vi "CRYAPI WSYSTEM.vi"(8 "sData":string, 9 "pVIF":refnum<vi>, 10 "sOption":string, 11 "sAction":string) -> (0 "bResult":bool=TRUE, 1 "pVIF_Out":refnum<vi>, 2 "sData_Out":string, 3 "tFrame_Out":T2)   [LabVIEW 2013]
uses:
  <vilib>/Utility/miscctls.llb/LVRectTypeDef.ctl
  CRYMain Sub Window Global.vi
panel:
  in  "nData":i32
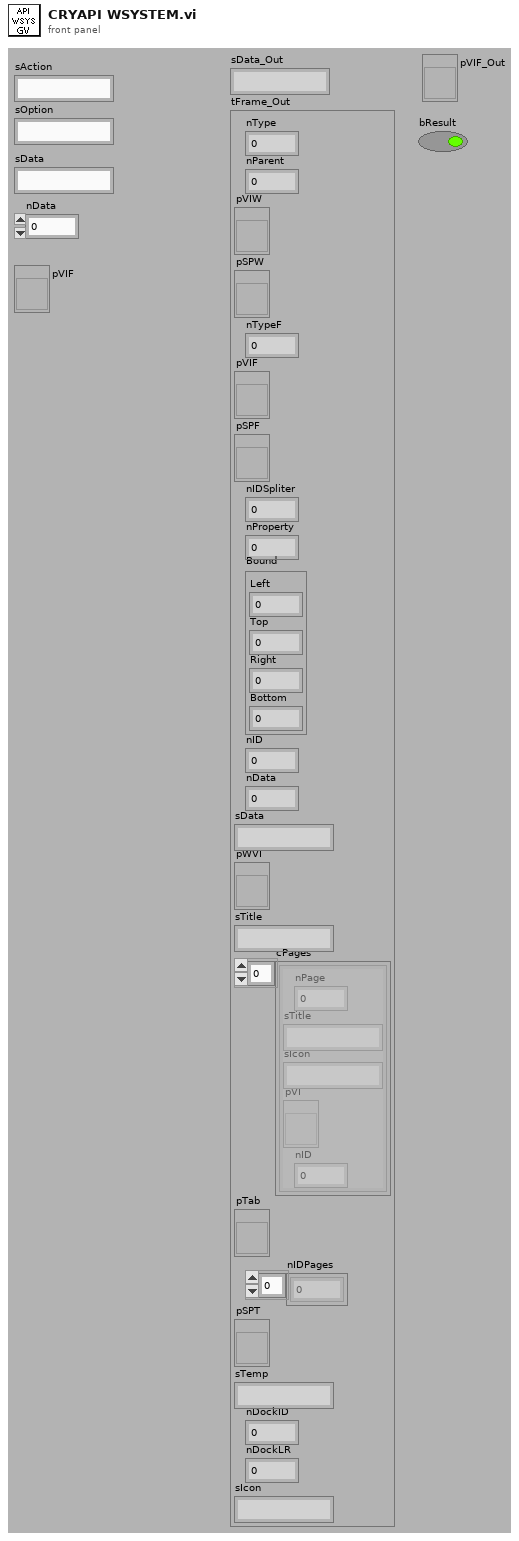
[diagram p1: front panel]
types:
  T1 = typedef "LVRectTypeDef.ctl" = cluster{"Left":i16, "Top":i16, "Right":i16, "Bottom":i16}
  T2 = cluster{"nType":i32, "nParent":i32, "pVIW":refnum<vi>, "pSPW":refnum<vi>, "nTypeF":i32, "pVIF":refnum<vi>, "pSPF":refnum<vi>, "nIDSpliter":i32, "nProperty":i32, "Bound":T1, "nID":i32, "nData":i32, "sData":string, "pWVI":refnum<vi>, "sTitle":string, "cPages":cluster{"nPage":i32, "sTitle":string, "sIcon":string, "pVI":refnum<vi>, "nID":i32}[], "pTab":refnum<vi>, "nIDPages":i32[], "pSPT":refnum<vi>, "sTemp":string, "nDockID":i32, "nDockLR":i32, "sIcon":string}
  T3 = cluster{"nData":i32, "sData":string, "sAction":string, "sOption":string}
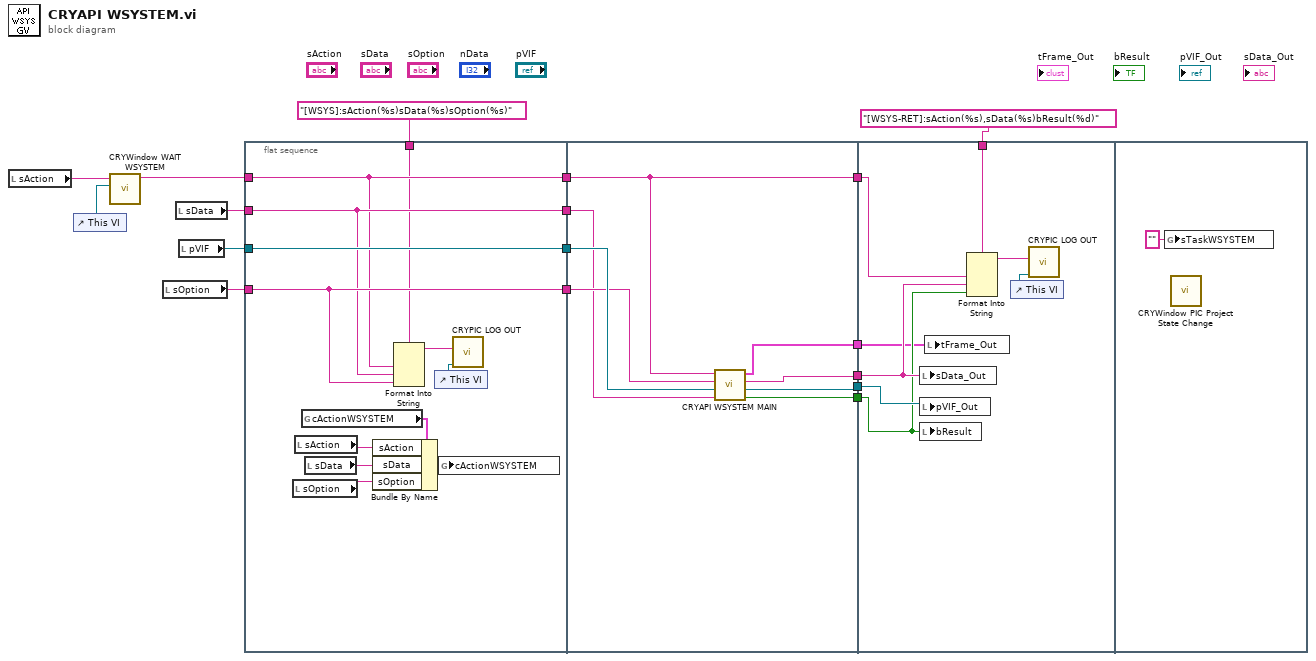
[diagram p0: block diagram]
diagram:
  n1 = local read "sAction"() -> (w13:string)
  n2 = control-ref of="This VI"() -> (w14:refnum<vi>)
  n3 = call "CRYWindow WAIT WSYSTEM.vi"("vi reference"=w14, "sAction"=w13) -> ("sAction_Out"=w12:string)  [unwired: 9 in]
  n4 = local read "sOption"() -> (w15:string)
  n5 = local read "sData"() -> (w17:string)
  n6 = local read "pVIF"() -> (w16:refnum<vi>)
  n7 = flat-sequence {
    tunnel: w12 -> [w19]
    tunnel: w17 -> [w20]
    tunnel: w16 -> [w22]
    tunnel: w15 -> [w21]
    tunnel: [w22] -> w11
    tunnel: [w21] -> w10
    tunnel: [w20] -> w9
    tunnel: [w19] -> w8
    tunnel: "[WSYS]:sAction(%s)sData(%s)sOption(%s)" ("format string") -> [w18]
    tunnel: w11 -> [w37]
    tunnel: w10 -> [w36]
    tunnel: w9 -> [w35]
    tunnel: w8 -> [w31]
    tunnel: [w34] -> w7
    tunnel: [w33] -> w6
    tunnel: [w32] -> w5
    tunnel: [w31] -> w4
    tunnel: [w30] -> w1
    tunnel: "[WSYS-RET]:sAction(%s),sData(%s)bResult(%d)" ("format string") -> [w44]
    tunnel: w7 -> [w41]
    tunnel: w6 -> [w43]
    tunnel: w5 -> [w40]
    tunnel: w4 -> [w42]
    tunnel: w1 -> [w38]
    frame #0 {
      n8 = local read "sOption"() -> (w27:string)
      n9 = local read "sAction"() -> (w29:string)
      n10 = global read "CRYMain Sub Window Global.vi" "cActionWSYSTEM"() -> (w25:T3)
      n11 = local read "sData"() -> (w28:string)
      n12 = Bundle By Name(cluster=w25, "sAction"=w29, "sData"=w28, "sOption"=w27) -> (w26:T3)
      n13 = Format Into String(format string=w18, w19, w20, w21) -> (resulting string=w24:string)  [unwired: 2 in, 1 out]
      n14 = control-ref of="This VI"() -> (w23:refnum<vi>)
      n15 = global write "CRYMain Sub Window Global.vi" "cActionWSYSTEM"(w26) -> ()
      n16 = call "CRYPIC LOG OUT.vi"("pVIRef"=w23, "sData"=w24) -> ()  [unwired: 10 in]
    }
    frame #1 {
      n17 = call "CRYAPI WSYSTEM MAIN.vi"("sData"=w35, "pVIF"=w37, "sOption"=w36, "sAction"=w31) -> ("bResult"=w32:bool, "pVIF_Out"=w33:refnum<vi>, "sData_Out"=w34:string, "tFrame_Out"=w30:T2)  [unwired: 4 in]
    }
    frame #2 {
      n18 = local write "sData_Out"(w41) -> ()
      n19 = local write "pVIF_Out"(w43) -> ()
      n20 = local write "bResult"(w40) -> ()
      n21 = local write "tFrame_Out"(w38) -> ()
      n22 = Format Into String(format string=w44, w42, w41, w40) -> (resulting string=w39:string)  [unwired: 2 in, 1 out]
      n23 = control-ref of="This VI"() -> (w45:refnum<vi>)
      n24 = call "CRYPIC LOG OUT.vi"("pVIRef"=w45, "sData"=w39) -> ()  [unwired: 10 in]
    }
    frame #3 {
      n25 = global write "CRYMain Sub Window Global.vi" "sTaskWSYSTEM"("" ("sTaskWSYSTEM")) -> ()
      n26 = call "CRYWindow PIC Project State Change.vi"() -> ()  [unwired: 12 in]
    }
  }
